vi "test.vi"() -> ()   [LabVIEW 2010]
uses:
  <vilib>/addons/Modulation/Analog/controls/Complex Data Waveform.ctl
  <vilib>/addons/Modulation/Digital/General/MT Generate Bits (Galois, PN Order).vi
  <vilib>/addons/Modulation/Digital/Impairments/Fading Profiles/MT Rician Fading Profile (Jakes).vi
  <vilib>/Analysis/2dsp.llb/Complex FFT.vi
  <vilib>/addons/Adaptive Filters/Create/AFT Create FIR LMS (Complex).vi
  <vilib>/addons/Adaptive Filters/Processing/AFT Filter Signal and Update Coefficients (Complex, Array).vi
  <vilib>/addons/Modulation/Digital/Impairments/Fading Profiles/MT Rayleigh Fading Profile (Jakes).vi
  <vilib>/imath/engines/lvmath2/RunTimeEngine/ErrorHandling/NIMS_Finalize Error.vi
  <vilib>/imath/engines/lvmath2/RunTimeEngine/Managers/WorkSpace/UID Generator.vi
  <vilib>/imath/engines/lvmath2/RunTimeEngine/Managers/SymbolTable/Clear UID.vi
  <vilib>/imath/engines/lvmath2/RunTimeEngine/NodeEndStatement/NIMS_NodeEndStatement_Output.vi
  <instcachedir>/0/NIMS_NodeEndStatement_Output_53EC0D466D134D7ABD903AC30B43404B.lvgen/NIMS_NodeEndStatement_Output_53EC0D466D134D7ABD903AC30B43404B_000.vi
  <vilib>/imath/engines/lvmath2/RunTimeEngine/BuiltInFunctions/length/NIMS_length(GV).vi
  <instcachedir>/0/NIMS_length(GV)_08A3D13377FD4E4B96F5795FBF3698FA.lvgen/NIMS_length(GV)_08A3D13377FD4E4B96F5795FBF3698FA_002.vi
  <vilib>/imath/engines/lvmath2/RunTimeEngine/RunTimeType/NIMS_RunTimeType_From StrictType (excl LVString).vi
  <vilib>/imath/engines/lvmath2/RunTimeEngine/LocalVariableDefStatement/MC_LocalVariableDefStatement_Display.vi
  <vilib>/imath/engines/lvmath2/RunTimeEngine/BuiltInFunctions/zeros/NIMS_V=zeros(I32,I32).vi
  <vilib>/imathl/engines/lvmath/Functions/Error Handling/Create Error.vi
  <vilib>/imath/engines/lvmath2/RunTimeEngine/RangeToken/NIMS_Range_R2 - Integer.vi
  <instcachedir>/0/NIMS_Range_R2 - Integer_217CA55F27D14E80B3D190635C7B3F47.lvgen/NIMS_Range_R2 - Integer_217CA55F27D14E80B3D190635C7B3F47_000.vi
  <vilib>/imath/engines/lvmath2/RunTimeEngine/CommandStatement/MC_CommandStatement_break.vi
  <vilib>/imath/engines/lvmath2/RunTimeEngine/VariableToken/Read/NIMS_Get Elements - RV(_) - Check.vi
  <instcachedir>/0/NIMS_Get Elements - RV(_) - Check_1F6F8656162345078B1D4DC9877DFAE9.lvgen/NIMS_Get Elements - RV(_) - Check_1F6F8656162345078B1D4DC9877DFAE9_004.vi
  <vilib>/imath/engines/lvmath2/RunTimeEngine/ReplaceToken/NIMS_Replace - Check Linear.vi
  <instcachedir>/0/NIMS_Replace - Check Linear_662D5651E4E34E0584DA82A256193A4C.lvgen/NIMS_Replace - Check Linear_662D5651E4E34E0584DA82A256193A4C_002.vi
  <vilib>/imath/engines/lvmath2/RunTimeEngine/ReplaceToken/NIMS_Replace - Size Check _(_)=S.vi
  <instcachedir>/0/NIMS_Replace - Size Check _(_)=S_6CAC13ACC74349C582FDAB09BCDAB70F.lvgen/NIMS_Replace - Size Check _(_)=S_6CAC13ACC74349C582FDAB09BCDAB70F_001.vi
  <vilib>/imath/engines/lvmath2/RunTimeEngine/ReplaceToken/NIMS_Replace - V(S)=S.vi
  <instcachedir>/0/NIMS_Replace - V(S)=S_78FDB6CCD265407D8926E4CF958018EB.lvgen/NIMS_Replace - V(S)=S_78FDB6CCD265407D8926E4CF958018EB_001.vi
  <vilib>/addons/Modulation/Digital/Impairments/MT Apply Flat Fading Profile.vi
  <vilib>/Analysis/2dsp.llb/Inverse Complex FFT.vi
  <vilib>/addons/Modulation/niDMT.lvlib
  <vilib>/Analysis/NI_AALPro.lvlib
  <vilib>/addons/Modulation/niAMT.lvlib
  <vilib>/imath/engines/lvmath2/RunTimeEngine/Managers/SymbolTable/NIMS_WorkSpace.lvlib
  <vilib>/addons/Adaptive Filters/NI_AdaptiveFilter.lvlib
panel:
  in  "布尔":bool
  out "TX Constellation":T1(graph)
  out "constellation graph":T2(graph)
  out "X":dbl[](graph)
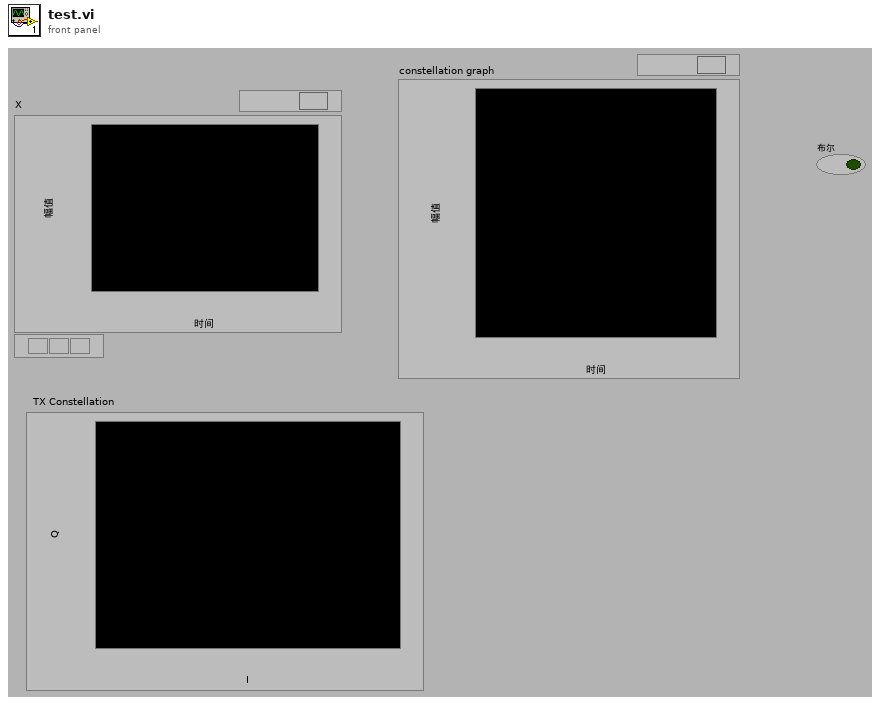
[diagram p1: front panel]
types:
  T1 = cluster{"Decimated Array":dbl[], "Decimated Array":dbl[]}[]
  T2 = cluster{"constellation":dbl[], "oversampled data":dbl[]}[]
  T3 = typedef "niAMT.lvlib/Complex Data Waveform.ctl" = cluster{"t0":dbl, "dt":dbl, "Y":cdb[]}
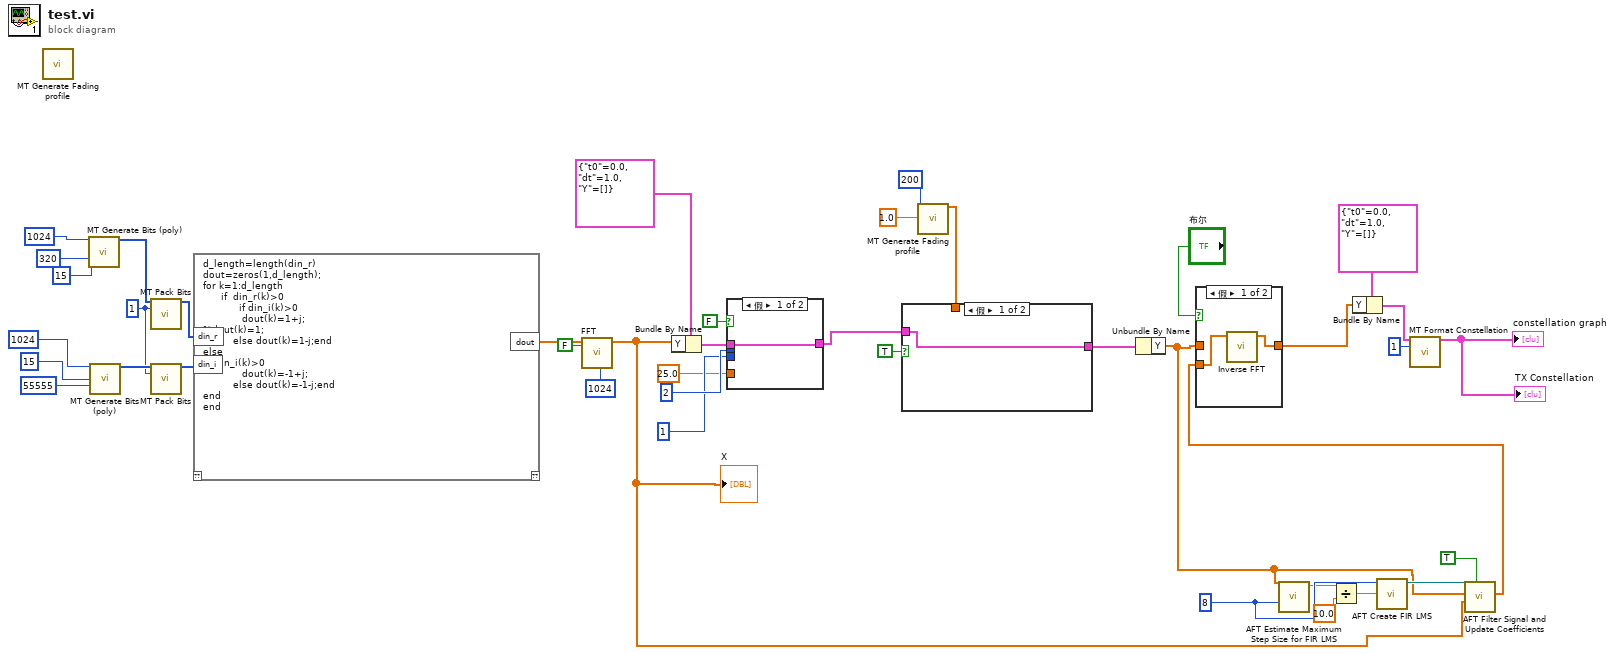
[diagram p0: block diagram]
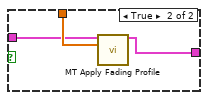
[diagram p2: hidden frame]
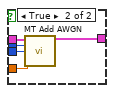
[diagram p3: hidden frame]
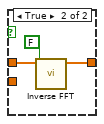
[diagram p4: hidden frame]
diagram:
  w19 = 8 ("filter length")
  w34 = 1 ("bits per integer")
  n1 = call-poly <vilib>:"MT Generate Fading profile.vi"() -> ()  [unwired: 13 in, 3 out]
  n2 = call-poly <vilib>:"MT Generate Bits (poly).vi"("total bits (128)"=1024, "PN sequence order (9)"=15, "seed in (0xD6BF7DF2)"=320) -> ("output bit stream"=w40:i8[])  [unwired: 10 in, 2 out]
  n3 = call-poly <vilib>:"MT Generate Bits (poly).vi"("total bits (128)"=1024, "PN sequence order (9)"=15, "seed in (0xD6BF7DF2)"=55555) -> ("output bit stream"=w36:i8[])  [unwired: 10 in, 2 out]
  n4 = call <vilib>:"MT Pack Bits.vi"("input bit stream"=w40, "bits per integer"=w34) -> ("output integers"=w31:i32[])  [unwired: 12 in, 1 out]
  n5 = call <vilib>:"MT Pack Bits.vi"("input bit stream"=w36, "bits per integer"=w34) -> ("output integers"=w32:i32[])  [unwired: 12 in, 1 out]
  n6 = mathscript code="d_length=length(din_r)\ndout=zeros(1,d_length);\nfor k=1:d_length\n      if  din_r(k)>0\n            if din_i(k)>0\n             dout(k)=1+j;\n%dout(k)=1;\n          else dout(k)=1-j;end\nelse   \n if din_i(k)>0\n             dout(k)=-1+j;\n          else dout(k)=-1-j;end\nend\nend"("din_r"=w31, "din_i"=w32) -> ("dout"=w15:cdb[])  [unwired: 1 in, 1 out]
  n7 = call-poly <vilib>:"FFT.vi"("FFT size"=1024, "shift?"=FALSE, "X"=w15) -> ("FFT {X}"=w1:cdb[])  [unwired: 7 in, 1 out]
  "X" <- w1
  n8 = Bundle By Name(cluster=T3 {"t0"=0.0, "dt"=1.0, "Y"=[]} ("input complex waveform"), "Y"=w1) -> (w28:T3)
  n9 = case shown="假" FALSE {
    tunnel: 2 ("samples per symbol (16)") -> [_ w47]
    tunnel: w28 -> [w42 w46]
    tunnel: 1 ("bits per symbol (1)") -> [_ w45]
    tunnel: 25.0 ("Eb/N0 (10 dB)") -> [_ w44]
    tunnel: [w42 w43] -> w8
    frame False {
    }
    frame True {
      n10 = call <vilib>:"MT Add AWGN.vi"("input complex waveform"=w46, "samples per symbol (16)"=w47, "bits per symbol (1)"=w45, "Eb/N0 (10 dB)"=w44) -> ("output complex waveform"=w43:T3)  [unwired: 9 in, 2 out]
    }
  }
  n11 = call-poly <vilib>:"MT Generate Fading profile.vi"("profile length (samples)"=200, "sampling frequency (Hz)"=1.0) -> ("fading profile"=w9:cdb[])  [unwired: 11 in, 2 out]
  n12 = case shown="假" TRUE {
    tunnel: w9 -> [_ w51]
    tunnel: w8 -> [w48 w50]
    tunnel: [w48 w49] -> w7
    frame False {
    }
    frame True {
      n13 = call-poly <vilib>:"MT Apply Fading Profile.vi"("input complex waveform"=w50, "fading profile"=w51) -> ("output complex waveform"=w49:T3)  [unwired: 12 in, 1 out]
    }
  }
  n14 = Unbundle By Name(w7) -> ("Y"=w5:cdb[])
  n15 = call <vilib>:"AFT Estimate Maximum Step Size for FIR LMS.vi"("filter length"=w19, "x(n)"=w5) -> ("maximum step size"=w3:dbl)  [unwired: 8 in, 1 out]
  n16 = Divide(x=w3, y=10.0) -> (x/y=w4:dbl)
  n17 = call-poly <vilib>:"AFT Create FIR LMS.vi"("step size"=w4, "filter length"=w19) -> ("adaptive filter out"=w18:refnum<k20>)  [unwired: 8 in, 1 out]
  n18 = call-poly <vilib>:"AFT Filter Signal and Update Coefficients.vi"("reset? (F)"=TRUE, "d(n)"=w1, "x(n)"=w5, "adaptive filter in"=w18) -> ("y(n)"=w14:cdb[])  [unwired: 4 in, 3 out]
  n19 = case shown="假" "布尔" {
    tunnel: [w52 w55] -> w16
    tunnel: w5 -> [_ w54]
    tunnel: w14 -> [w53 _]
    frame False {
      n20 = call-poly <vilib>:"Inverse FFT.vi"("FFT {X}"=w53) -> ("X"=w52:cdb[])  [unwired: 9 in, 1 out]
    }
    frame True {
      n21 = call-poly <vilib>:"Inverse FFT.vi"("shift?"=FALSE, "FFT {X}"=w54) -> ("X"=w55:cdb[])  [unwired: 8 in, 1 out]
    }
  }
  n22 = Bundle By Name(cluster=T3 {"t0"=0.0, "dt"=1.0, "Y"=[]} ("waveform"), "Y"=w16) -> (w23:T3)
  n23 = call <vilib>:"MT Format Constellation.vi"("waveform"=w23, "samples per symbol"=1) -> ("constellation graph"=→"constellation graph" →"TX Constellation":T2)  [unwired: 12 in, 1 out]
